vi "asset.create.request.vi"(8 "error in":errorcluster, 10 "Description":string, 11 "Title":string) -> (0 "error out":errorcluster, 3 "request":string)   [LabVIEW 2020, in "Nominal Client.lvclass"]
uses:
  Nominal Client.lvclass
  23b81bce-5bf5-4553-8ece-e154542c4e39.vi
  b8348f26-5a24-4650-bd02-6cd2d99a680c.vi
  <vilib>/JDP Science/JSONtext/Variant to JSON Text.vi
  <vilib>/JDP Science/JSONtext/LVClass Serializer/JSONtext LVClass Serializer.lvclass
  <vilib>/JDP Science/JSONtext/JSONtext.lvlib
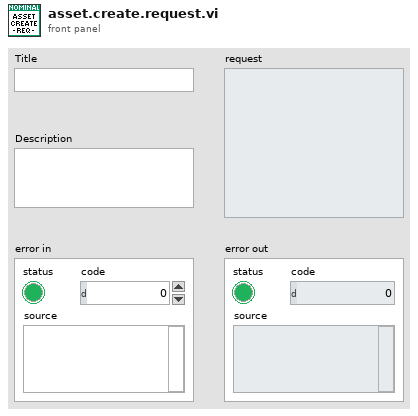
[diagram p1: front panel]
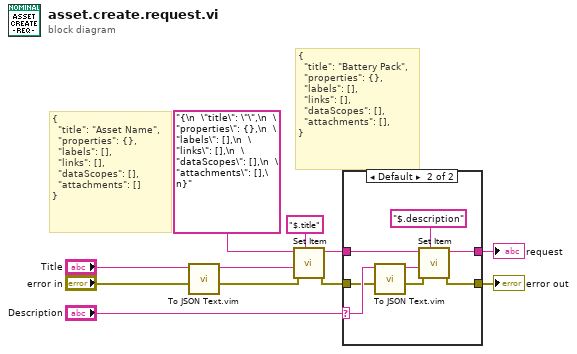
[diagram p0: block diagram]
diagram:
  # "{\n  \"title\": \"Battery Pack\",\n  \"properties\": {},\n  \"labels\": [],\n  \"links\": [],\n  \"dataScopes\": [],\n  \"attachments\": [],\n}"
  # "{\n  \"title\": \"Asset Name\",\n  \"properties\": {},\n  \"labels\": [],\n  \"links\": [],\n  \"dataScopes\": [],\n  \"attachments\": []\n}"
  n1 = call "To JSON Text.vim"("error in (no error)"="error in", "Anything"="Title") -> ("error out"=w7:errorcluster, "<JSON>"=w9:string)  [unwired: 8 in]
  n2 = call <vilib>:"Set Item.vi"("$Path or Item Name"="$.title", "error in (no error)"=w7, "JSON to Insert"=w9, "JSON"="{\n  \"title\": \"\",\n  \"properties\": {},\n  \"labels\": [],\n  \"links\": [],\n  \"dataScopes\": [],\n  \"attachments\": [],\n}") -> ("error out"=w6:errorcluster, "<JSON>"=w8:string)  [unwired: 4 in, 1 out]
  n3 = case shown="Default" "Description" {
    selector: "Description" -> [_ w19]
    tunnel: w8 -> [w13 w20]
    tunnel: [w13 w17] -> w1
    tunnel: w6 -> [w12 w16]
    tunnel: [w12 w14] -> w2
    frame "" {
    }
    frame Default {
      n4 = call "To JSON Text.vim"("error in (no error)"=w16, "Anything"=w19) -> ("error out"=w15:errorcluster, "<JSON>"=w18:string)  [unwired: 8 in]
      n5 = call <vilib>:"Set Item.vi"("$Path or Item Name"="$.description", "error in (no error)"=w15, "JSON to Insert"=w18, "JSON"=w20) -> ("error out"=w14:errorcluster, "<JSON>"=w17:string)  [unwired: 4 in, 1 out]
    }
  }
  "error out" <- w2
  "request" <- w1
